vi "Cell 3D Measurement.vi"(10 "Serial Number":string="1234", 11 "Part Number":string="B0CG1KL3RC") -> (2 "Diameter":dbl=18.0, 3 "Length":dbl=65.0)   [LabVIEW 2021]
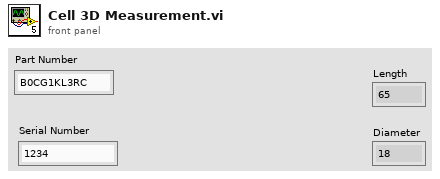
[diagram p1: front panel]
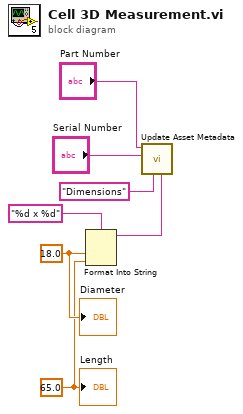
[diagram p0: block diagram]
diagram:
  w3 = 18.0 ("Width")
  w2 = 65.0 ("Length")
  n1 = Format Into String(format string="%d x %d", w3, w2) -> (resulting string=w1:string)  [unwired: 2 in, 1 out]
  n2 = call "Update Asset Metadata.vi"("Value"=w1, "Property"="Dimensions", "Serial Number"="Serial Number", "Part Number"="Part Number") -> ()  [unwired: 6 in, 2 out]
  "Length" <- w2
  "Diameter" <- w3
